vi "6.vi"() -> ()   [LabVIEW 2017, in "ErrorStructureDrawer-Tests.lvlib"]
uses:
  ErrorStructureDrawer/Controls/ErrorControlType.ctl
  ErrorStructureDrawer-Tests.lvlib
  ErrorStructureDrawer/ErrorStructureDrawer.lvlib
panel:
  out "Error control type":T1
  out "Default control style found?":bool
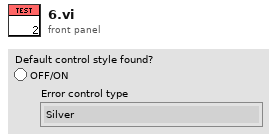
[diagram p1: front panel]
types:
  T1 = typedef "ErrorStructureDrawer.lvlib/ErrorControlType.ctl" = enum16{"Silver", "Modern", "Classic", "LabVIEW default"}
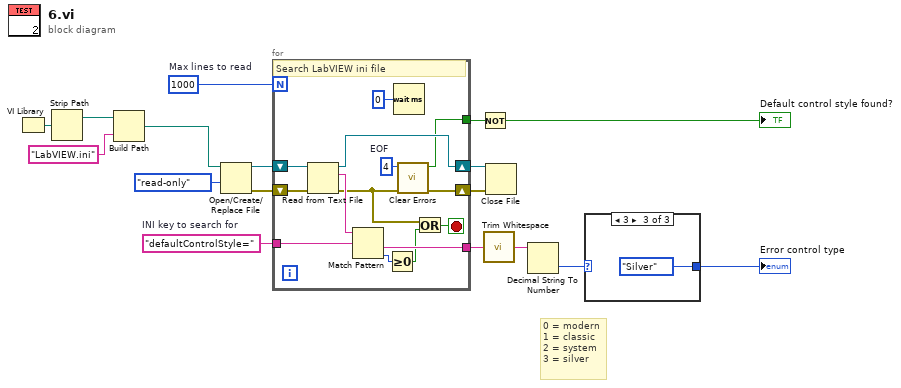
[diagram p0: block diagram]
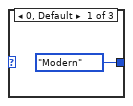
[diagram p2: hidden frame]
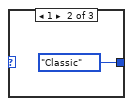
[diagram p3: hidden frame]
diagram:
  w7 = "defaultControlStyle="  # INI key to search for
  w8 = 1000  # Max lines to read
  # "0 = modern\n1 = classic\n2 = system\n3 = silver"
  n1 = VI Library() -> (path=w17:path)
  n2 = Strip Path(path=w17) -> (stripped path=w16:path)  [unwired: 1 out]
  n3 = Build Path(base path=w16, name or relative path="LabVIEW.ini") -> (appended path=w14:path)
  n4 = Open/Create/Replace File(file path (use dialog)=w14, access (0:read/write)=enum16{"read/write", "read-only", "write-only"}."read-only") -> (refnum out=w12:refnum<file>, error out=w11:errorcluster)  [unwired: 4 in, 1 out]
  n5 = for {
    N: w8 -> [_]
    shift-right: [w29] -> w9
    shift-left: w12 -> [w31]
    shift-right: [w28] -> w10
    shift-left: w11 -> [w30]
    tunnel: [w27] -> w4
    tunnel: w7 -> [w24]
    tunnel: [w23] -> w6
    stop <- w19 stop-if-true
    w18 = 4  # EOF
    # "Search LabVIEW ini file"
    n6 = Read from Text File(file (use dialog)=w31, error in=w30) -> (refnum out=w29:refnum<file>, text=w25:string, error out=w21:errorcluster)  [unwired: 2 in, 1 out]
    n7 = Match Pattern(string=w25, regular expression=w24) -> (after substring=w23:string, offset past match=w22:i32)  [unwired: 1 in, 2 out]
    n8 = Greater Or Equal To 0?(x=w22) -> (x >= 0?=w20:bool)
    n9 = Wait (ms)(milliseconds to wait=u32 0) -> ()  [unwired: 1 out]
    n10 = call <vilib>:"Clear Errors.vi"("error in (no error)"=w21, "specific error code to clear (0: all)"=w18) -> ("error out"=w28:errorcluster, "specific error cleared?"=w27:bool)  [unwired: 4 in]
    n11 = Or(x=w21, y=w20) -> (x .or. y?=w19:bool)
  }
  n12 = Not(x=w4) -> (.not. x?=→"Default control style found?":bool)
  n13 = call <vilib>:"Trim Whitespace.vi"("string"=w6) -> ("trimmed string"=w5:string)  [unwired: 1 in]
  n14 = Close File(refnum=w9, error in=w10) -> ()  [unwired: 2 out]
  n15 = Decimal String To Number(string=w5) -> (number=w2:i32)  [unwired: 2 in, 1 out]
  n16 = case shown="3" w2 {
    tunnel: [ErrorControlType."Modern" ("Error control type") ErrorControlType."Classic" ("Error control type") ErrorControlType."Silver" ("Error control type")] -> w1
    frame 0, Default {
    }
    frame 1 {
    }
    frame 3 {
    }
  }
  "Error control type" <- w1
